vi "Tektronix AFG 3000 Series Waveform Burst.vi"() -> ()   [LabVIEW 2019]
doc: "Demonstrates how to configure burst mode and trigger source.\n\nNote:\n\nFor external trigger source an external trigger input would be required."
uses:
  <userlib>/Tektronix AFG 3000 Series/Tektronix AFG 3000 Series.lvlib
panel:
  in  "Burst Mode (0: Triggered)":u16(ring) items=["Triggered", "Gated"]
  in  "Channel (0: Channel 1)":u16(ring) items=["Channel 1", "Channel 2"]
  in  "Internal Trigger Rate (500)":dbl=500.0
  in  "Burst Count (5)":i32=5
  in  "VISA resource name":refnum<visa-resource-name>
  # "(c) 2006-2012 National Instruments.  ALL RIGHTS RESERVED."
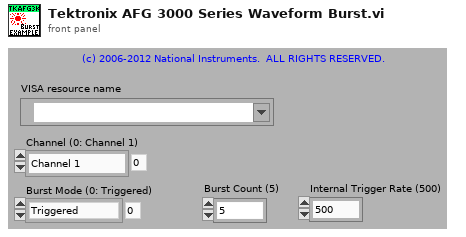
[diagram p1: front panel]
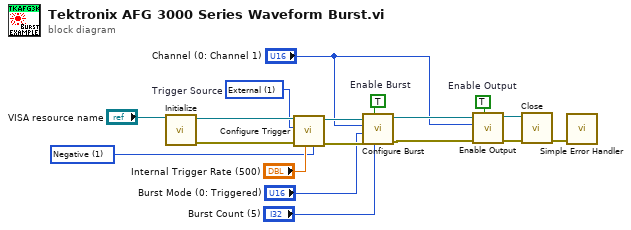
[diagram p0: block diagram]
diagram:
  w1 = u16 1 items=["Positive", "Negative"] ("External Trigger Slope (0: Positive)")
  w3 = u16 1 items=["Internal"=3, "External"=1]  # Trigger Source
  w8 = TRUE  # Enable Output
  w9 = TRUE  # Enable Burst
  n1 = call <userlib>:"Initialize.vi"("VISA resource name"="VISA resource name") -> ("error out"=w4:errorcluster, "VISA resource name out"=w5:refnum<visa-resource-name>)  [unwired: 9 in]
  n2 = call <userlib>:"Configure Trigger.vi"("External Trigger Slope (0: Positive)"=w1, "Internal Trigger Rate (500)"="Internal Trigger Rate (500)", "error in (no error)"=w4, "Trigger Source (3:Internal)"=w3, "VISA resource name"=w5) -> ("error out"=w18:errorcluster, "VISA resource name out"=w17:refnum<visa-resource-name>)  [unwired: 5 in]
  n3 = call <userlib>:"Configure Burst.vi"("Burst Count (5)"="Burst Count (5)", "Enable Burst (T: Enable)"=w9, "error in (no error)"=w18, "Burst Mode (0: Triggered)"="Burst Mode (0: Triggered)", "Channel (0: Channel 1)"="Channel (0: Channel 1)", "VISA resource name"=w17) -> ("error out"=w15:errorcluster, "VISA resource name out"=w16:refnum<visa-resource-name>)  [unwired: 4 in]
  n4 = call <userlib>:"Enable Output.vi"("Enable Output (T: Enable)"=w8, "error in (no error)"=w15, "Channel (0: Channel 1)"="Channel (0: Channel 1)", "VISA resource name"=w16) -> ("error out"=w13:errorcluster, "VISA resource name out"=w14:refnum<visa-resource-name>)  [unwired: 5 in]
  n5 = call <userlib>:"Close.vi"("error in (no error)"=w13, "VISA resource name"=w14) -> ("error out"=w12:errorcluster)  [unwired: 9 in]
  n6 = call <vilib>:"Simple Error Handler.vi"("error in (no error)"=w12) -> ()  [unwired: 4 in, 5 out]
